vi "loadDataNodeBegin.vi"(8 "error in (no error)":errorcluster, 10 "XML Refnum in":refnum<file>, 11 "Channel in":refnum<class "Parameter.lvclass">) -> (0 "error out":errorcluster, 2 "XML Refnum out":refnum<file>, 3 "Channel out":refnum<class "Parameter.lvclass">)   [LabVIEW 2013, in "Parameter.lvclass"]
doc: "Part of the file loading process. Occurs at the beginning of a node being loaded. Loads the common xceDataNode data name and description."
uses:
  Parameter.lvclass
  Parameter.lvclass/Parameter.ctl
  xCE/xceDataNode/xceDataNode.lvclass
  XML Parser/XML Parser.lvclass
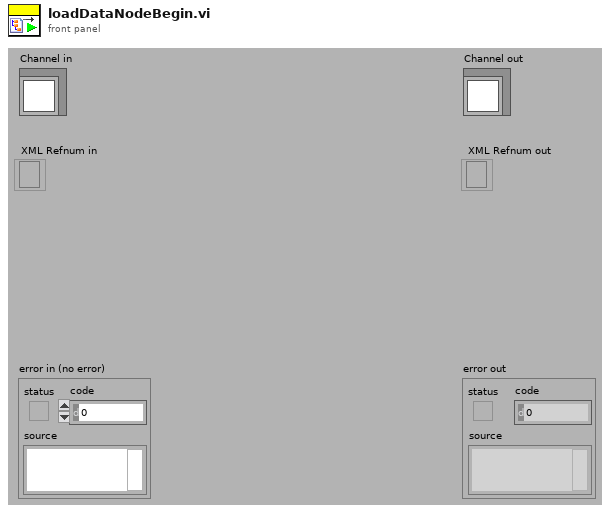
[diagram p1: front panel]
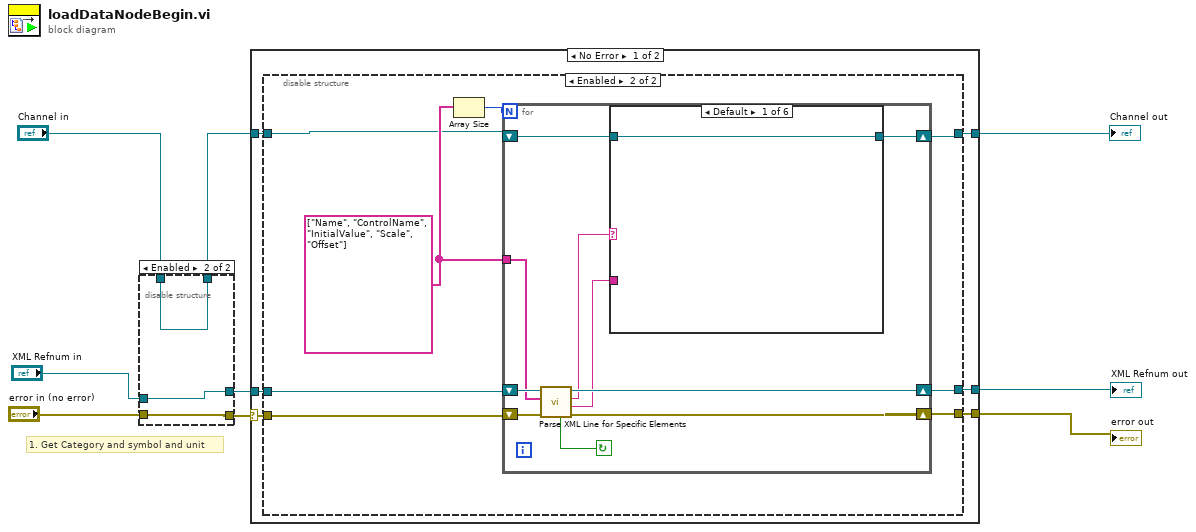
[diagram p0: block diagram]
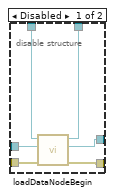
[diagram p2: hidden frame]
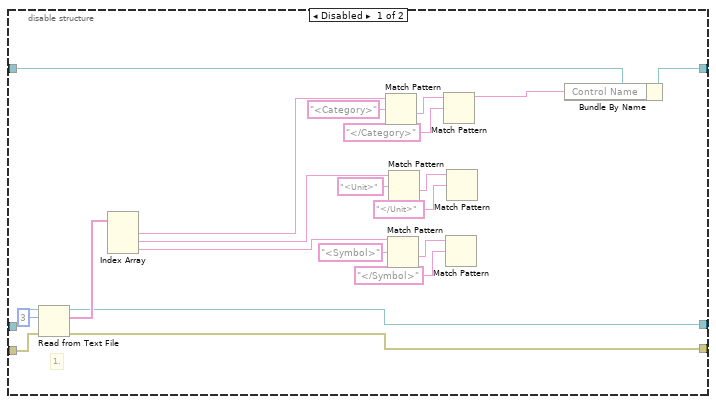
[diagram p3: hidden frame]
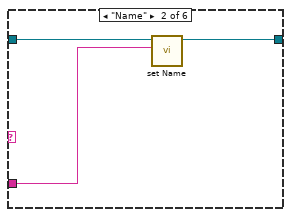
[diagram p4: hidden frame]
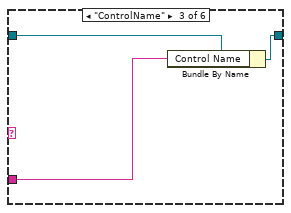
[diagram p5: hidden frame]
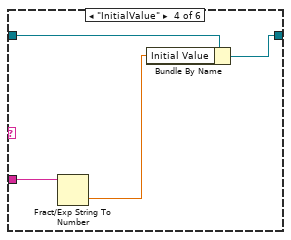
[diagram p6: hidden frame]
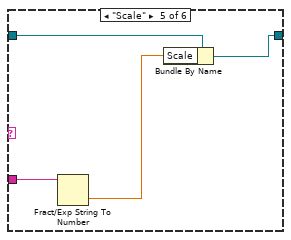
[diagram p7: hidden frame]
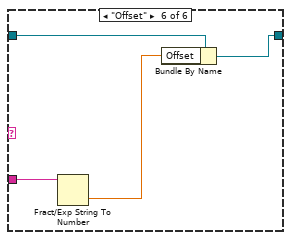
[diagram p8: hidden frame]
diagram:
  # "1. Get Category and symbol and unit"
  n1 = disable-structure shown="Enabled" {
    disable-tunnel: [w15 w16] -> w6
    disable-tunnel: "error in (no error)" -> [w14 w16]
    disable-tunnel: "XML Refnum in" -> [w13 w17]
    disable-tunnel: [w12 w17] -> w3
    disable-tunnel: "Channel in" -> [w11 w18]
    disable-tunnel: [w10 w18] -> w1
    frame Disabled {
      n2 = call-parent "loadDataNodeBegin.vi"("error in (no error)"=w14, "XML Refnum in"=w13, "xceDataNode in"=w11) -> ("error out"=w15:errorcluster, "XML Refnum out"=w12:refnum<file>, "xceDataNode out"=w10:refnum<class "Parameter.lvclass">)  [unwired: 6 in]
    }
    frame Enabled {
    }
  }
  n3 = case shown="No Error" w6 {
    selector: w6 -> [w24 w85]
    tunnel: [w22 w85] -> w7
    tunnel: [w20 w83] -> w9
    tunnel: w3 -> [w23 w84]
    tunnel: [w21 w84] -> w8
    tunnel: w1 -> [w19 w83]
    frame No Error {
      n4 = disable-structure shown="Enabled" {
        disable-tunnel: w24 -> [w45 w49]
        disable-tunnel: w23 -> [w44 w50]
        disable-tunnel: [w41 w47] -> w22
        disable-tunnel: [w39 w48] -> w21
        disable-tunnel: [w38 w46] -> w20
        disable-tunnel: w19 -> [w37 w51]
        frame Disabled {
          # "1."
          n5 = Read from Text File(file (use dialog)=w44, count=3, error in=w45) -> (refnum out=w39:refnum<file>, text=w42:string[], error out=w41:errorcluster)  [unwired: 1 in, 1 out]
          n6 = Index Array(array=w42) -> (element #1=w40:string, element #2=w25:string, element #3=w26:string)  [unwired: 3 in]
          n7 = Match Pattern(string=w40, regular expression="<Category>") -> (after substring=w35:string)  [unwired: 1 in, 3 out]
          n8 = Match Pattern(string=w26, regular expression="<Symbol>") -> (after substring=w31:string)  [unwired: 1 in, 3 out]
          n9 = Match Pattern(string=w25, regular expression="<Unit>") -> (after substring=w28:string)  [unwired: 1 in, 3 out]
          n10 = Match Pattern(string=w35, regular expression="</Category>") -> (before substring=w33:string)  [unwired: 1 in, 3 out]
          n11 = Match Pattern(string=w31, regular expression="</Symbol>") -> ()  [unwired: 1 in, 4 out]
          n12 = Match Pattern(string=w28, regular expression="</Unit>") -> ()  [unwired: 1 in, 4 out]
          n13 = Bundle By Name(cluster=w37, "Control Name"=w33) -> (w38:refnum<class "Parameter.lvclass">)
        }
        frame Enabled {
          w53 = string[] ["Name", "ControlName", "InitialValue", "Scale", "Offset"] ("Token List")
          n14 = Array Size(array=w53) -> (size(s)=w52:i32)
          n15 = for {
            N: w52 -> [_]
            shift-right: [w61] -> w48
            shift-left: w50 -> [w63]
            shift-right: [w60] -> w47
            shift-left: w49 -> [w62]
            shift-right: [w54] -> w46
            shift-left: w51 -> [w55]
            tunnel: w53 -> [w59]
            stop <- w58 continue-if-true
            n16 = call "Parse XML Line for Specific Elements.vi"("error in (no error)"=w62, "Elements"=w59, "XML Refnum in"=w63) -> ("error out"=w60:errorcluster, "Value"=w56:string, "Element Name"=w57:string, "XML Refnum out"=w61:refnum<file>, "Element Found"=w58:bool)  [unwired: 4 in]
            n17 = case shown="Default" w57 {
              tunnel: w56 -> [_ w65 w68 w72 w76 w80]
              tunnel: w55 -> [w64 w67 w70 w74 w78 w82]
              tunnel: [w64 w66 w69 w73 w77 w81] -> w54
              frame Default {
              }
              frame "Name" {
                n18 = call "set Name.vi"("Name"=w65, "xceDataNode in"=w67) -> ("xceDataNode out"=w66:refnum<class "Parameter.lvclass">)  [unwired: 8 in, 1 out]
              }
              frame "ControlName" {
                n19 = Bundle By Name(cluster=w70, "Control Name"=w68) -> (w69:refnum<class "Parameter.lvclass">)
              }
              frame "InitialValue" {
                n20 = Fract/Exp String To Number(string=w72) -> (number=w71:dbl)  [unwired: 3 in, 1 out]
                n21 = Bundle By Name(cluster=w74, "Initial Value"=w71) -> (w73:refnum<class "Parameter.lvclass">)
              }
              frame "Scale" {
                n22 = Fract/Exp String To Number(string=w76) -> (number=w75:dbl)  [unwired: 3 in, 1 out]
                n23 = Bundle By Name(cluster=w78, "Scale"=w75) -> (w77:refnum<class "Parameter.lvclass">)
              }
              frame "Offset" {
                n24 = Fract/Exp String To Number(string=w80) -> (number=w79:dbl)  [unwired: 3 in, 1 out]
                n25 = Bundle By Name(cluster=w82, "Offset"=w79) -> (w81:refnum<class "Parameter.lvclass">)
              }
            }
          }
        }
      }
    }
    frame Error {
    }
  }
  "error out" <- w7
  "Channel out" <- w9
  "XML Refnum out" <- w8
